vi "3ph Power Main (SubVI).vi"(8 "error in (no error)":errorcluster) -> (0 "error out":errorcluster)   [LabVIEW 2019]
uses:
  3ph Inputs.ctl
  Globals and Definitions/Initialization Globals.vi
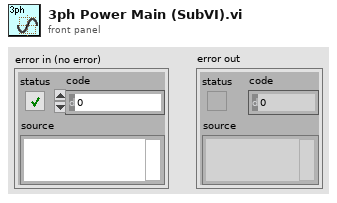
[diagram p1: front panel]
types:
  T1 = typedef "3ph Inputs.ctl" = cluster{"voltage channels":tag, "minimum voltage value":dbl, "maximum voltage value":dbl, "3ph sample rate [Hz]":dbl, "3phf samples per channel":i32, "Voltage Scaling":dbl, "Current Scaling":dbl}
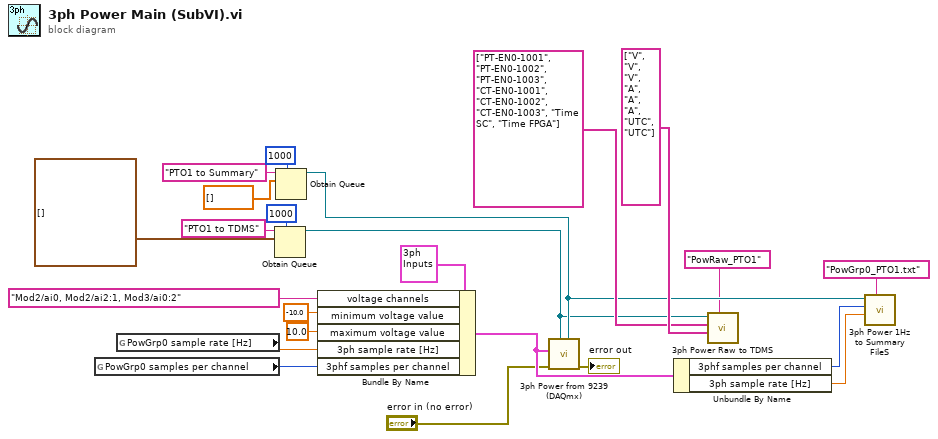
[diagram p0: block diagram]
diagram:
  n1 = global read "Initialization Globals.vi" "PowGrp0 samples per channel"() -> (w16:i32)
  n2 = global read "Initialization Globals.vi" "PowGrp0 sample rate [Hz]"() -> (w17:dbl)
  n3 = Obtain Queue(max queue size (-1, unlimited)=1000, name (unnamed)="PTO1 to TDMS", element data type=waveform(dbl)[] [] ("data")) -> (queue out=w1:refnum<queue>)  [unwired: 2 in, 2 out]
  n4 = Obtain Queue(max queue size (-1, unlimited)=1000, name (unnamed)="PTO1 to Summary", element data type=dbl[] [] ("appended array")) -> (queue out=w10:refnum<queue>)  [unwired: 2 in, 2 out]
  n5 = Bundle By Name(cluster=T1 {"voltage channels"="Mod3/ai0:2", "minimum voltage value"=-10.0, "maximum voltage value"=10.0, "3ph sample rate [Hz]"=5000.0, "3phf samples per channel"=500, "Voltage Scaling"=100.0, "Current Scaling"=100.0} ("3ph Inputs"), "voltage channels"=tag "Mod2/ai0, Mod2/ai2:1, Mod3/ai0:2", "minimum voltage value"=-10.0, "maximum voltage value"=10.0, "3ph sample rate [Hz]"=w17, "3phf samples per channel"=w16) -> (w19:T1)
  n6 = call "3ph Power from 9239 (DAQmx).vi"("PTO1 Summary"=w10, "PTO1 TDMS"=w1, "error in"="error in (no error)", "3ph Inputs"=w19) -> ("error out"=→"error out":errorcluster)  [unwired: 7 in]
  n7 = Unbundle By Name(w19) -> ("3phf samples per channel"=w7:i32, "3ph sample rate [Hz]"=w6:dbl)
  n8 = call "3ph Power Raw to TDMS.vi"("PowRaw Name"="PowRaw_PTO1", "Channel Units"=string[] ["V", "V", "V", "A", "A", "A", "UTC", "UTC"], "Channel Names"=string[] ["PT-EN0-1001", "PT-EN0-1002", "PT-EN0-1003", "CT-EN0-1001", "CT-EN0-1002", "CT-EN0-1003", "Time SC", "Time FPGA"], "Queue in wfm"=w1) -> ()  [unwired: 8 in]
  n9 = call "3ph Power 1Hz to Summary FileS.vi"("1Hz Filename"="PowGrp0_PTO1.txt", "3ph sample rate [Hz]"=w6, "3phf samples per channel"=w7, "Queue in"=w10) -> ()  [unwired: 8 in]
